vi "Convert Array from ImprocOptions.vi"(1 "IMPROCOPTIONS":T1 {"FilterCode" items=["PREWITT_3X3_V"=1, "PREWITT_3X3_H"=2, "SOBEL_3X3_V"=3, "SOBEL_3X3_H"=4, "LAPLACIAN_3X3"=5, "LAPLACIAN_5X5"=6, "GAUSSIAN_3X3"=7, "GAUSSIAN_5X5"=8, "HIPASS_3x3"=9, "HIPASS_5x5"=10, "SHARPEN_3X3"=11, "USERFILTER"=-1]; "Rotate" min=-90 max=90 step=1; "Saturation" min=-100 max=100 step=1; "Contrast" min=-100 max=100 step=1; "Bright" min=-100 max=100 step=1}) -> (0 "Array":i32[](array[numeric]))   [LabVIEW 2013, in "VRI.lvlib"]
uses:
  VRI.lvlib
  _Type Defs/PhInt IMPROCOPTIONS.ctl
  _Type Defs/PhInt WBGAIN.ctl
  _Type Defs/FilterCode.ctl
  _Type Defs/IMFILTER.ctl
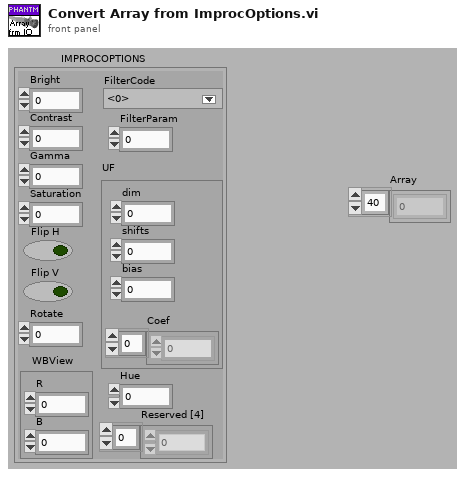
[diagram p1: front panel]
types:
  T1 = typedef "VRI.lvlib/PhInt IMPROCOPTIONS.ctl" = cluster{"Bright":i32, "Contrast":i32, "Gamma":sgl, "Saturation":i32, "Flip H":bool, "Flip V":bool, "Rotate":i32, "WBView":T2, "FilterCode":T3, "FilterParam":i32, "UF":T4, "Hue":i32, "Reserved [4]":i32[]}
  T2 = typedef "VRI.lvlib/PhInt WBGAIN.ctl" = cluster{"R":sgl, "B":sgl}
  T3 = typedef "VRI.lvlib/FilterCode.ctl" = i32
  T4 = typedef "VRI.lvlib/IMFILTER.ctl" = cluster{"dim":i32, "shifts":i32, "bias":i32, "Coef":i32[]}
  T5 = cluster{"Bright":i32, "Contrast":i32, "Bright":i32, "Saturation":i32, i32, i32, "Rotate":i32}
  T6 = cluster{"FilterCode":T3, "FilterParam":i32, "dim":i32, "shifts":i32, "bias":i32}
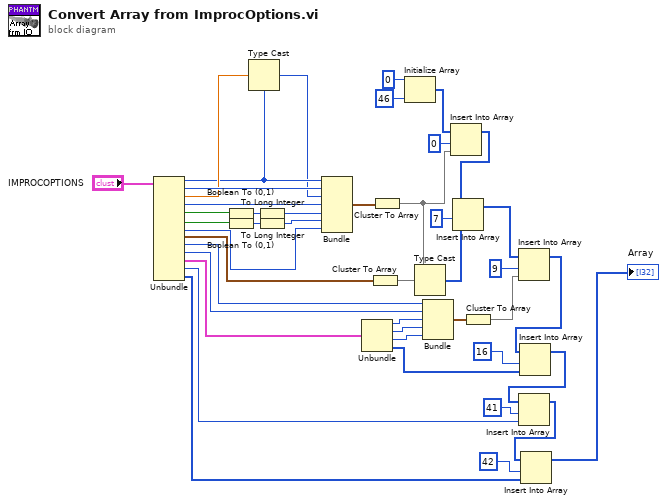
[diagram p0: block diagram]
diagram:
  n1 = Unbundle("IMPROCOPTIONS") -> ("Bright"=w35:i32, "Contrast"=w42:i32, "Gamma"=w36:sgl, "Saturation"=w37:i32, "Flip H"=w41:bool, "Flip V"=w39:bool, "Rotate"=w31:i32, "WBView"=w29:T2, "FilterCode"=w28:T3, "FilterParam"=w27:i32, "UF"=w43:T4, "Hue"=w7:i32, "Reserved [4]"=w5:i32[])
  n2 = Boolean To (0,1)(Boolean=w41) -> (0, 1=w40:i16)
  n3 = Boolean To (0,1)(Boolean=w39) -> (0, 1=w38:i16)
  n4 = Type Cast(type=w35, x=w36) -> (*(type *) &x=w34:i32)
  n5 = To Long Integer(number=w40) -> (32bit integer=w33:i32)
  n6 = To Long Integer(number=w38) -> (32bit integer=w32:i32)
  n7 = Bundle("Bright"=w35, "Contrast"=w42, "Bright"=w34, "Saturation"=w37, w33, w32, "Rotate"=w31) -> (w30:T5)  [unwired: 1 out]
  n8 = Unbundle(w43) -> ("dim"=w26:i32, "shifts"=w25:i32, "bias"=w24:i32, "Coef"=w15:i32[])
  n9 = Cluster To Array(cluster=w29) -> (array=w23:sgl[])
  n10 = Cluster To Array(cluster=w30) -> (array=w9:i32[])
  n11 = Initialize Array(0 ("element"), 46 ("dimension size")) -> (w11:i32[])
  n12 = Type Cast(type=w9, x=w23) -> (*(type *) &x=w22:i32[])
  n13 = Bundle("FilterCode"=w28, "FilterParam"=w27, "dim"=w26, "shifts"=w25, "bias"=w24) -> (w18:T6)  [unwired: 1 out]
  n14 = Insert Into Array(array=w11, index=0, new element=w9) -> (w8:i32[])
  n15 = Insert Into Array(array=w8, index=7, new element=w22) -> (w20:i32[])
  n16 = Cluster To Array(cluster=w18) -> (array=w17:T3[])
  n17 = Insert Into Array(array=w20, index=9, new element=w17) -> (w16:i32[])
  n18 = Insert Into Array(array=w16, index=16, new element=w15) -> (w2:i32[])
  n19 = Insert Into Array(array=w2, index=41, new element=w7) -> (w1:i32[])
  n20 = Insert Into Array(array=w1, index=42, new element=w5) -> (→"Array":i32[])
